vi "Clear Accurate Measure Time Out.vi"(7 "ESP32 ref":refnum<visa-resource-name>="COM4", 8 "error in (no error)":errorcluster, 11 "DMM ref":refnum<visa-resource-name>) -> (0 "error out":errorcluster, 1 "error?":bool, 2 "Time out count":i32, 3 "VISA Refnum out":refnum<visa-resource-name>)   [LabVIEW 2023]
uses:
  <vilib>/Utility/error.llb/DialogType.ctl
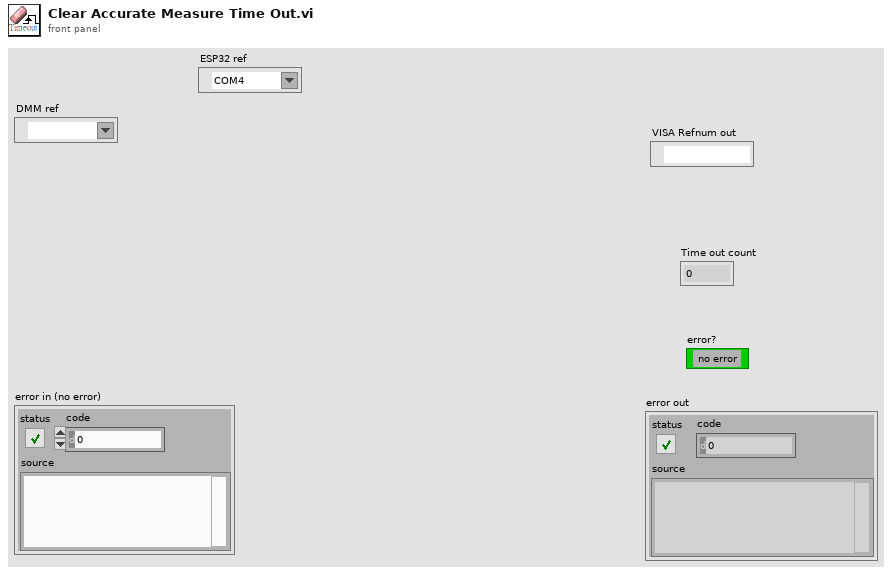
[diagram p1: front panel]
types:
  T1 = typedef "DialogType.ctl" = u16
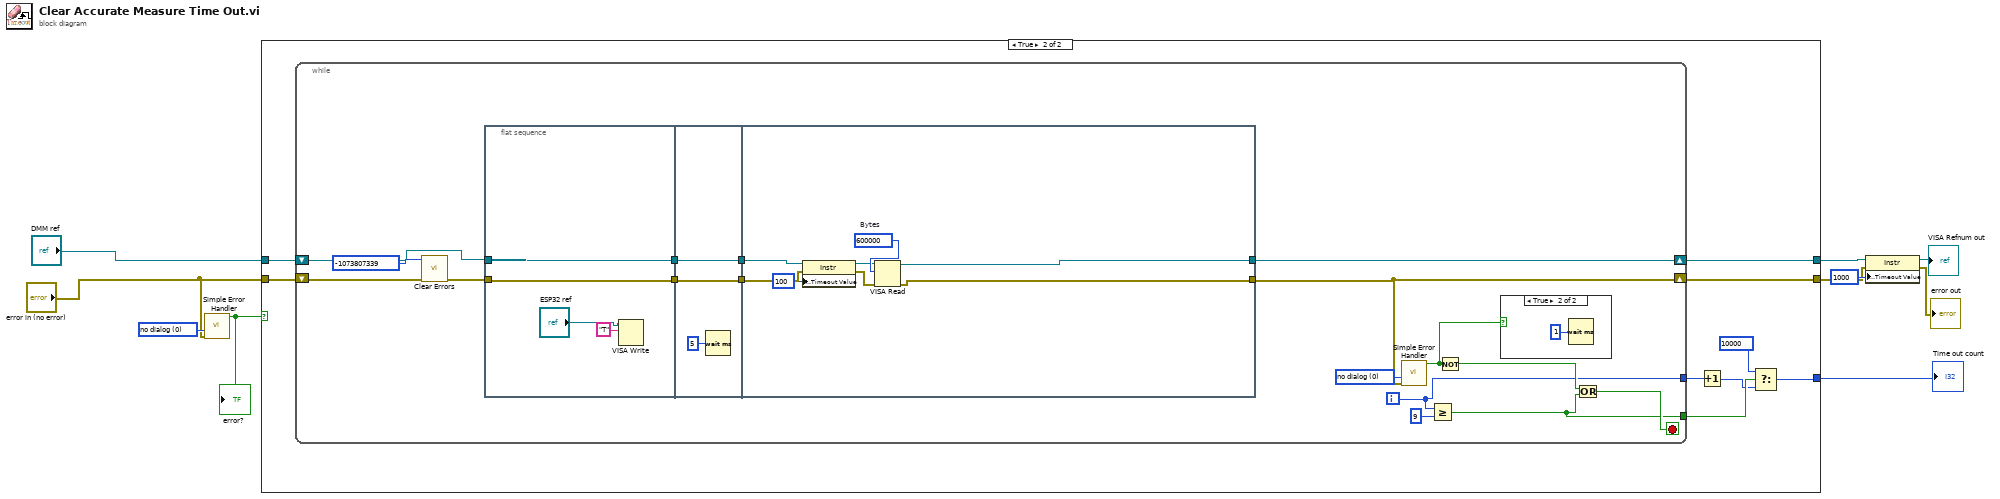
[diagram p0: block diagram]
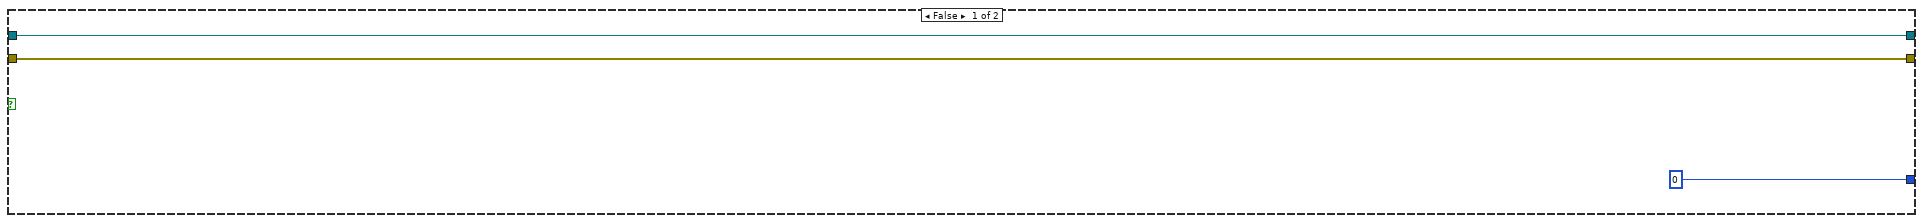
[diagram p2: hidden frame]
diagram:
  w9 = T1 0 items=["no dialog", "OK message", "continue or stop message", "OK message + warnings", "continue/stop + warnings"] ("type of dialog (OK msg:1)")
  n1 = call <vilib>:"Simple Error Handler.vi"("type of dialog (OK msg:1)"=w9, "error in (no error)"="error in (no error)") -> ("error?"=w7:bool)  [unwired: 3 in, 4 out]
  "error?" <- w7
  n2 = case shown="True" w7 {
    tunnel: [w13 w22] -> w4
    tunnel: "error in (no error)" -> [w12 w21]
    tunnel: "DMM ref" -> [w13 w20]
    tunnel: [w12 w19] -> w3
    tunnel: [0 w16] -> w6
    frame False {
    }
    frame True {
      n3 = while {
        shift-right: [w33] -> w19
        shift-left: w21 -> [w37]
        shift-right: [w39] -> w22
        shift-left: w20 -> [w35]
        tunnel: [w29] -> w15
        tunnel: [w28] -> w18
        i -> [w29]
        stop <- w30 stop-if-true
        w34 = T1 0 items=["no dialog", "OK message", "continue or stop message", "OK message + warnings", "continue/stop + warnings"] ("type of dialog (OK msg:1)")
        n4 = call <vilib>:"Clear Errors.vi"("error in (no error)"=w37, "specific error code to clear (0: all)"=-1073807339 ("code out")) -> ("error out"=w36:errorcluster)  [unwired: 4 in, 1 out]
        n5 = flat-sequence {
          tunnel: w36 -> [w43]
          tunnel: w35 -> [w44]
          tunnel: [w44] -> w24
          tunnel: [w43] -> w26
          tunnel: w26 -> [w47]
          tunnel: [w47] -> w25
          tunnel: w24 -> [w46]
          tunnel: [w46] -> w23
          tunnel: [w54] -> w33
          tunnel: [w55] -> w39
          tunnel: w23 -> [w52]
          tunnel: w25 -> [w50]
          frame #0 {
            n6 = VISA Write(VISA resource name="ESP32 ref", write buffer="T") -> ()  [unwired: 1 in, 3 out]
          }
          frame #1 {
            n7 = Wait (ms)(milliseconds to wait=u32 5) -> ()  [unwired: 1 out]
          }
          frame #2 {
            w53 = u32 600000  # Bytes
            n8 = property class="Instr"(reference=w52, error in=w50, "General Settings:Timeout Value"=u32 100) -> (reference out=w51:refnum<visa-resource-name>, error out=w49:errorcluster)
            n9 = VISA Read(VISA resource name=w51, byte count=w53, error in (no error)=w49) -> (VISA resource name out=w55:refnum<visa-resource-name>, error out=w54:errorcluster)  [unwired: 2 out]
          }
        }
        n10 = call <vilib>:"Simple Error Handler.vi"("type of dialog (OK msg:1)"=w34, "error in (no error)"=w33) -> ("error?"=w27:bool)  [unwired: 3 in, 4 out]
        n11 = Greater Or Equal?(x=w29, y=9) -> (x >= y?=w28:bool)
        n12 = Not(x=w27) -> (.not. x?=w31:bool)
        n13 = case shown="True" w27 {
          frame False {
          }
          frame True {
            n14 = Wait (ms)(milliseconds to wait=u32 1) -> ()  [unwired: 1 out]
          }
        }
        n15 = Or(x=w31, y=w28) -> (x .or. y?=w30:bool)
      }
      n16 = Increment(x=w15) -> (x+1=w14:i32)
      n17 = Select(t=10000, s=w18, f=w14) -> (s? t:f=w16:i32)
    }
  }
  "Time out count" <- w6
  n18 = property class="Instr"(reference=w4, error in=w3, "General Settings:Timeout Value"=u32 1000) -> (reference out=→"VISA Refnum out":refnum<visa-resource-name>, error out=→"error out":errorcluster)
